vi "CloseFile.vi"(8 "error in (no error)":errorcluster, 11 "INIFileClass in":refnum<class "INIFileClass.lvclass">) -> (0 "error out":errorcluster, 2 "AllKeysFound":bool, 3 "INIFileClass out":refnum<class "INIFileClass.lvclass">)   [LabVIEW 2013, in "INIFileClass.lvclass"]
uses:
  INIFileClass.lvclass
  INIFileClass.lvclass/INIFileClass.ctl
  <vilib>/Utility/config.llb/NI_LVConfig.lvlib
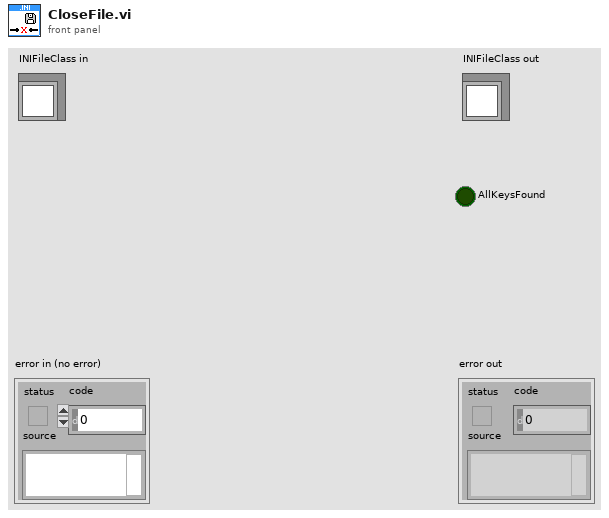
[diagram p1: front panel]
types:
  T1 = typedef "NI_LVConfig.lvlib/Config Data RefNum.ctl" = refnum<k1>
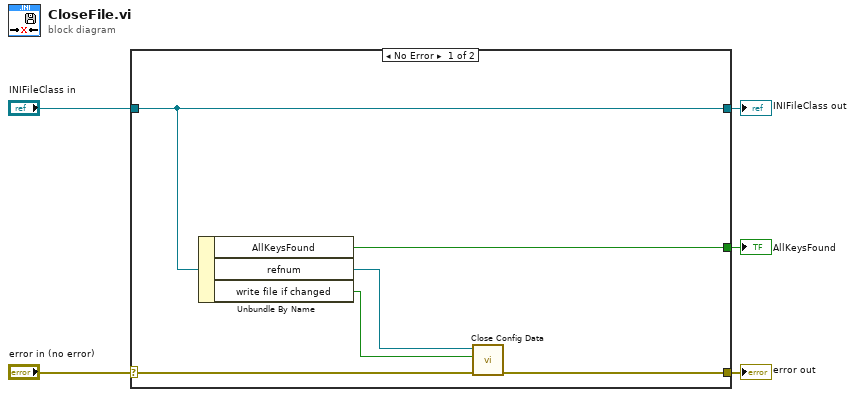
[diagram p0: block diagram]
diagram:
  n1 = case shown="No Error" "error in (no error)" {
    selector: "error in (no error)" -> [w11 w13]
    tunnel: [w10 w13] -> w4
    tunnel: [w8 w12] -> w2
    tunnel: "INIFileClass in" -> [w8 w12]
    tunnel: [w6 _] -> w1
    frame No Error {
      n2 = Unbundle By Name(w8) -> ("AllKeysFound"=w6:bool, "refnum"=w9:T1, "write file if changed"=w7:bool)
      n3 = call <vilib>:"Close Config Data.vi"("error in (no error)"=w11, "write file if changed (T)"=w7, "refnum"=w9) -> ("error out"=w10:errorcluster)  [unwired: 7 in, 1 out]
    }
    frame Error {
    }
  }
  "error out" <- w4
  "INIFileClass out" <- w2
  "AllKeysFound" <- w1
